vi "ROIEdges.vi"(0 "Array Subset":T1, 1 "reduce pts by factor of":i32=4, 2 "raw x coord":dbl[][](array[numeric]) format="%.2f", 3 "raw y coord":dbl[][](array[numeric]) format="%.2f", 4 "no oversample?":bool) -> (5 "x box":dbl[][](array[numeric]) format="%.2f", 6 "y box":dbl[][](array[numeric]) format="%.2f")   [LabVIEW 2022 SP3]
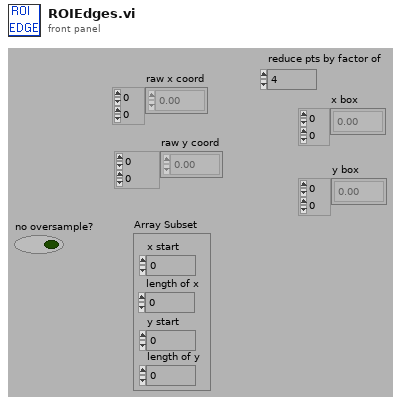
[diagram p1: front panel]
types:
  T1 = cluster{"x start":i32, "length of x":i32, "y start":i32, "length of y":i32}
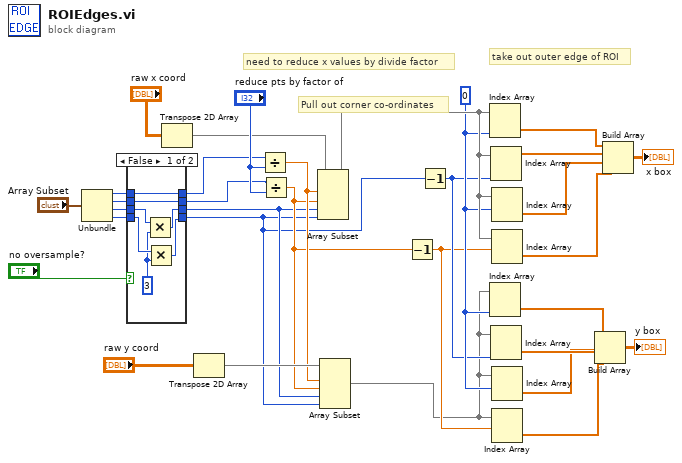
[diagram p0: block diagram]
diagram:
  w29 = 0 ("Disabled Index")
  # "need to reduce x values by divide factor"
  # "take out outer edge of ROI"
  # "Pull out corner co-ordinates"
  n1 = Unbundle("Array Subset") -> ("x start"=w15:i32, "length of x"=w13:i32, "y start"=w11:i32, "length of y"=w10:i32)
  n2 = case shown="False" "no oversample?" {
    tunnel: [w39 w43] -> w14
    tunnel: w15 -> [w39 w43]
    tunnel: [w38 w42] -> w12
    tunnel: w13 -> [w38 w42]
    tunnel: [w34 w41] -> w3
    tunnel: w11 -> [w37 w41]
    tunnel: [w35 w40] -> w2
    tunnel: w10 -> [w36 w40]
    frame False {
      w33 = 3
      n3 = Multiply(x=w37, y=w33) -> (x*y=w34:i32)
      n4 = Multiply(x=w36, y=w33) -> (x*y=w35:i32)
    }
    frame True {
    }
  }
  n5 = Transpose 2D Array(2D array="raw x coord") -> (transposed array=w8:dbl[][])
  n6 = Transpose 2D Array(2D array="raw y coord") -> (transposed array=w7:dbl[][])
  n7 = Divide(x=w14, y="reduce pts by factor of") -> (x/y=w5:dbl)
  n8 = Divide(x=w12, y="reduce pts by factor of") -> (x/y=w4:dbl)
  n9 = Array Subset(array=w8, index (row)=w5, length (row)=w4, index (col)=w3, length (col)=w2) -> (w30:dbl[][])
  n10 = Array Subset(array=w7, index (row)=w5, length (row)=w4, index (col)=w3, length (col)=w2) -> (w1:dbl[][])
  n11 = Decrement(x=w4) -> (x-1=w27:dbl)
  n12 = Decrement(x=w2) -> (x-1=w28:i32)
  n13 = Index Array(array=w30, index (col)=w29) -> (element=w26:dbl[])  [unwired: 1 in]
  n14 = Index Array(array=w1, index (col)=w29) -> (element=w21:dbl[])  [unwired: 1 in]
  n15 = Index Array(array=w30, index (col)=w28) -> (element=w25:dbl[])  [unwired: 1 in]
  n16 = Index Array(array=w1, index (col)=w28) -> (element=w20:dbl[])  [unwired: 1 in]
  n17 = Index Array(array=w30, index (row)=w29) -> (element=w24:dbl[])  [unwired: 1 in]
  n18 = Index Array(array=w30, index (row)=w27) -> (element=w23:dbl[])  [unwired: 1 in]
  n19 = Index Array(array=w1, index (row)=w29) -> (element=w19:dbl[])  [unwired: 1 in]
  n20 = Index Array(array=w1, index (row)=w27) -> (element=w18:dbl[])  [unwired: 1 in]
  n21 = Build Array(w21, w20, w19, w18) -> (→"y box":dbl[][])
  n22 = Build Array(w26, w25, w24, w23) -> (→"x box":dbl[][])
